vi "DBconnectiontest2.vi"() -> ()   [LabVIEW 2019]
uses:
  <vilib>/addons/database/Auxilliary.llb/DB Tools DataTypes.ctl
  <vilib>/addons/database/Connection.llb/DB Tools Open Connec (String).vi
  <vilib>/addons/database/NI_Database_API.lvlib
panel:
  in  "index":i32=1
  out "column information":T2(array[cluster])=[{"name"="assemble_Tray", "database data type"=enum."Long (I32)", "defined size"=1}, {"name"="screw_A_Tray", "database data type"=enum."Long (I32)", "defined size"=1}, {"name"="screw_B_Tray", "database data type"=enum."Long (I32)", "defined size"=1}]
  out "columns":string[](array[string])=["assemble_Tray", "screw_A_Tray", "screw_B_Tray"]
  out "error out":errorcluster
  out "tables":string[](array[string])=["glue_data", "preparation", "production_record", "workplace_data", "trace_xe_action_map", "trace_xe_event_map"]
  in  "DBlink":string="Driver={ODBC Driver 17 for SQL Server};Server=localhost\\SQLEXPRESS;Database=ZDX201;UID=labview;PWD=Dsa@54137926"
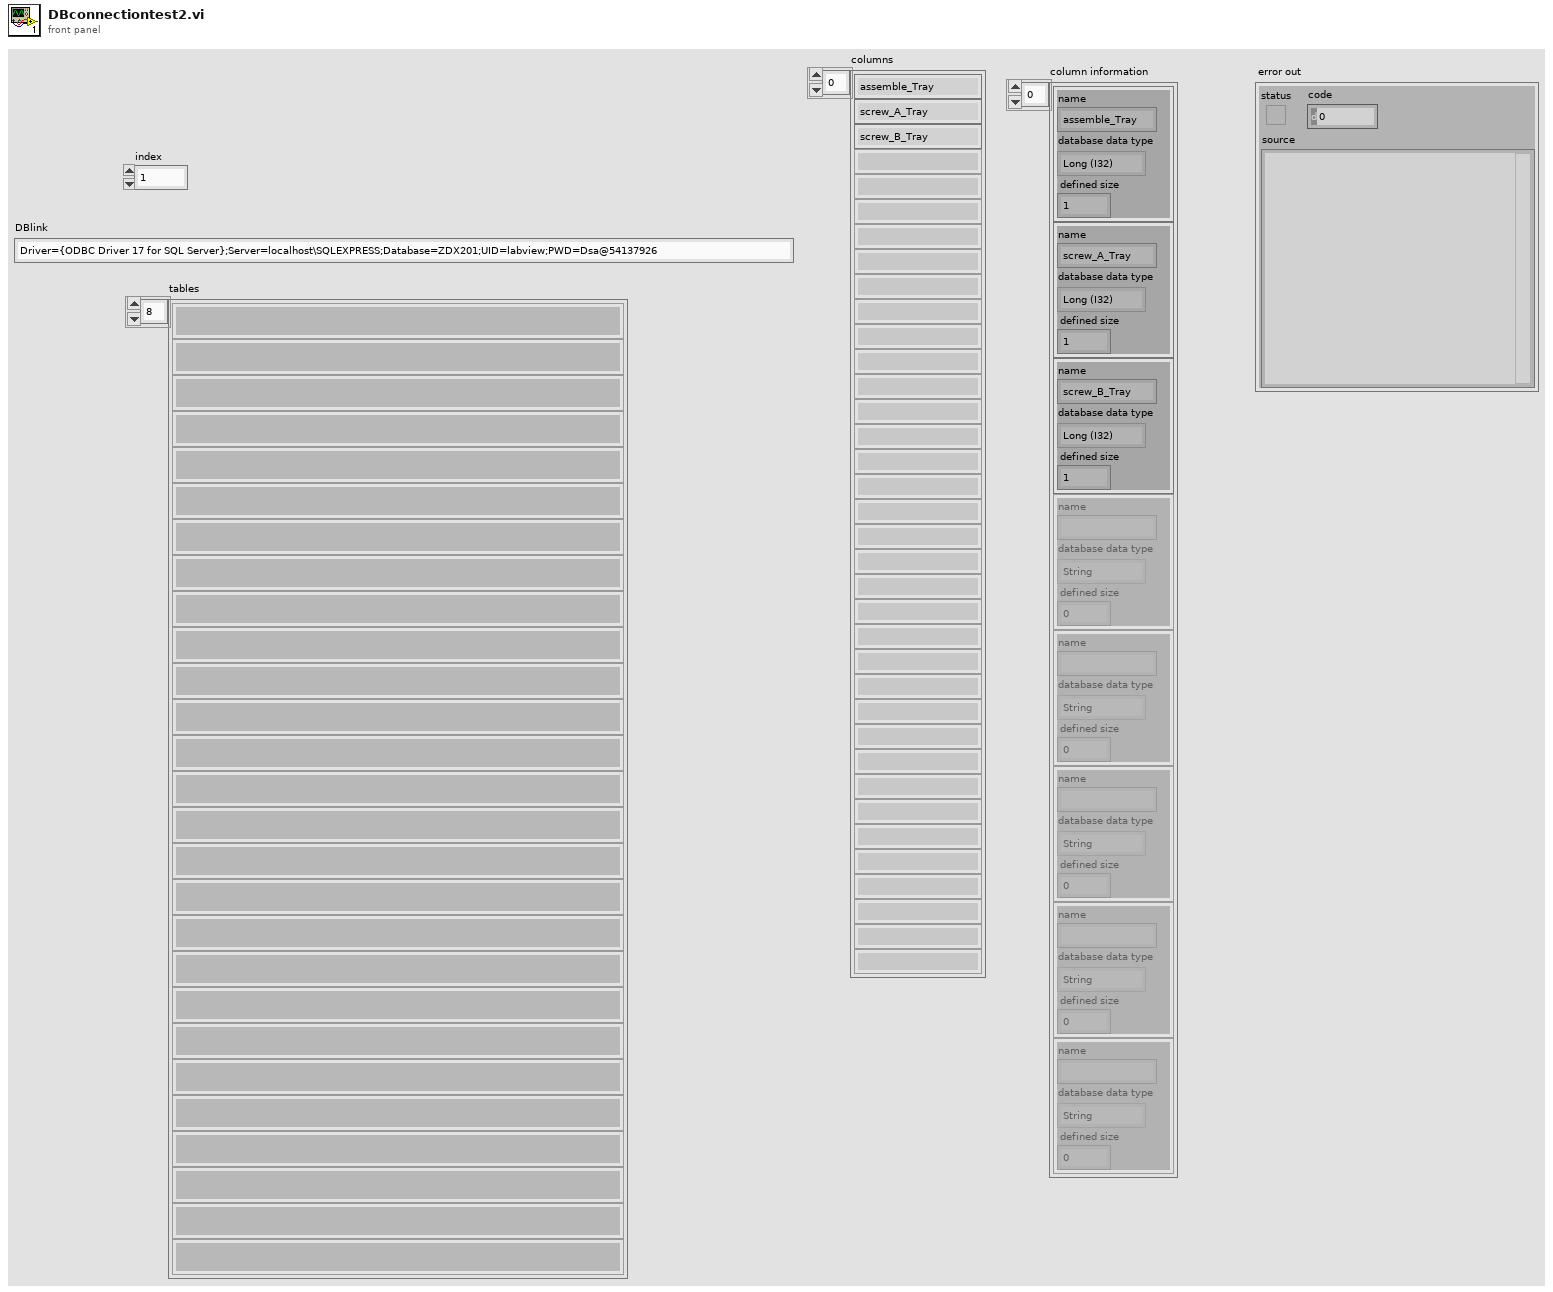
[diagram p1: front panel]
types:
  T1 = typedef "NI_Database_API.lvlib/DB Tools DataTypes.ctl" = enum16{"String", "Long (I32)", "Single (SGL)", "Double (DBL)", "Date/Time", "Binary"}
  T2 = cluster{"name":string, "database data type":T1, "defined size":i32}[]
  T3 = typedef "NI_Database_API.lvlib/Conn ObjectReference.ctl" = refnum<k1>
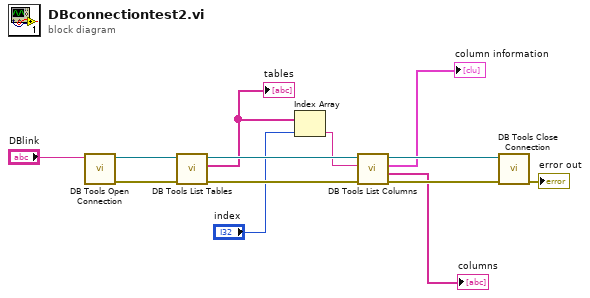
[diagram p0: block diagram]
diagram:
  n1 = call-poly <vilib>:"DB Tools Open Connection.vi"("connection information"="DBlink") -> ("error out"=w11:errorcluster, "connection reference"=w12:T3)  [unwired: 7 in]
  n2 = call <vilib>:"DB Tools List Tables.vi"("error in (no error)"=w11, "connection reference"=w12) -> ("error out"=w7:errorcluster, "tables"=w3:string[], "connection reference out"=w9:T3)  [unwired: 3 in]
  "tables" <- w3
  n3 = Index Array(array=w3, index="index") -> (element=w1:string)
  n4 = call <vilib>:"DB Tools List Columns.vi"("error in (no error)"=w7, "table"=w1, "connection reference"=w9) -> ("error out"=w6:errorcluster, "columns"=→"columns":string[], "column information"=→"column information":T2, "connection reference out"=w8:T3)  [unwired: 1 in]
  n5 = call <vilib>:"DB Tools Close Connection.vi"("error in (no error)"=w6, "connection reference"=w8) -> ("error out"=→"error out":errorcluster)  [unwired: 5 in]
